vi "LOC subReadWriteVIStringINIKeys(Boolean).vi"(4 "Mode":enum16{"Read", "Write"}(ring), 5 "Section":string, 6 "error in (no error)":errorcluster, 8 "ConfigFileRefnum":T1, 9 "ControlRefnum":refnum<vi>) -> (0 "error out":errorcluster)   [LabVIEW 2020, in "Localization_Tools.lvlib"]
uses:
  Localization_Tools.lvlib
  <vilib>/Utility/config.llb/Config Data RefNum.ctl
  <vilib>/Utility/config.llb/NI_LVConfig.lvlib
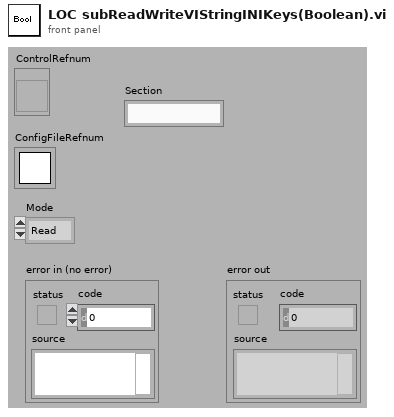
[diagram p1: front panel]
types:
  T1 = typedef "NI_LVConfig.lvlib/Config Data RefNum.ctl" = refnum<k1>
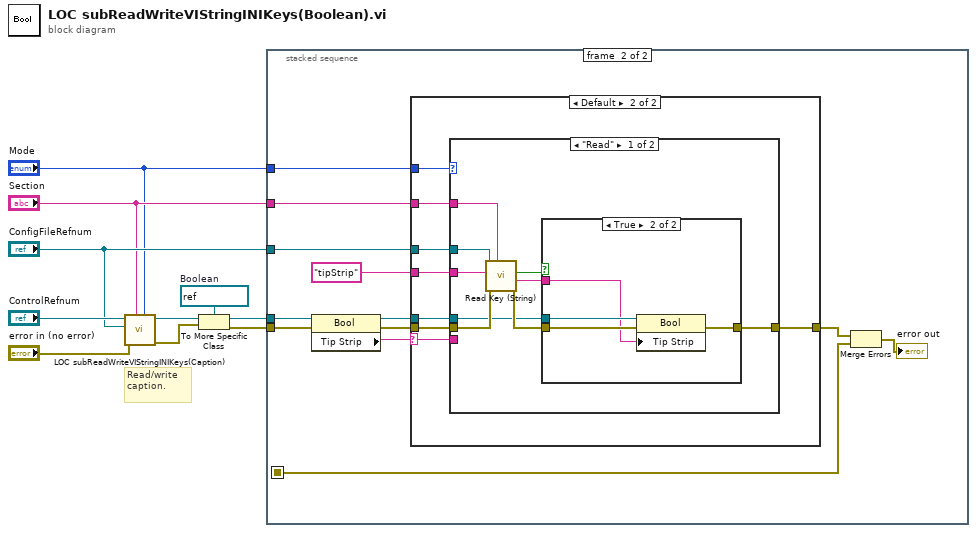
[diagram p0: block diagram]
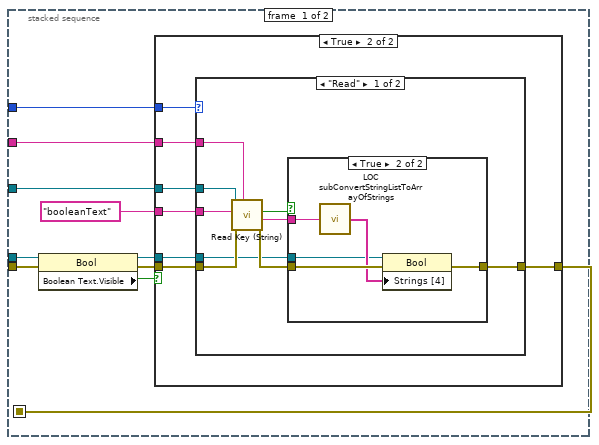
[diagram p2: hidden frame]
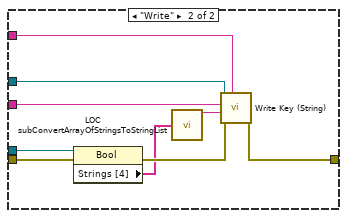
[diagram p5: hidden frame]
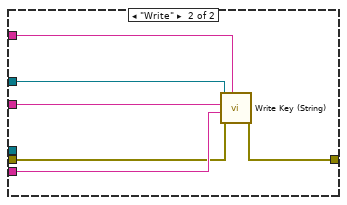
[diagram p8: hidden frame]
diagram:
  w5 = refnum<vi> refnum  # Boolean
  # "Read/write\ncaption."
  n1 = call "LOC subReadWriteVIStringINIKeys(Caption).vi"("Mode"="Mode", "Section"="Section", "error in (no error)"="error in (no error)", "ConfigFileRefnum"="ConfigFileRefnum", "ControlRefnum"="ControlRefnum") -> ("error out"=w3:errorcluster, "dup ControlRefnum"=w4:refnum<vi>)  [unwired: 3 in]
  n2 = To More Specific Class(target class=w5, reference=w4, error in=w3) -> (specific class reference=w2:refnum<vi>, error out=w1:errorcluster)
  n3 = stacked-sequence {
    seq-local: [w12 _] -> [_ w54]
    tunnel: "ConfigFileRefnum" -> [w20 w64]
    tunnel: "Section" -> [w19 w63]
    tunnel: "Mode" -> [w18 w62]
    tunnel: w2 -> [w15 w61]
    tunnel: w1 -> [w14 w60]
    frame #0 {
      n4 = property class="Bool"(reference=w15, error in=w14) -> (reference out=w17:refnum<vi>, error out=w16:errorcluster, "Boolean Text.Visible"=w13:bool)
      n5 = case shown="True" w13 {
        tunnel: "booleanText" ("key") -> [_ w28]
        tunnel: w20 -> [_ w27]
        tunnel: w19 -> [_ w26]
        tunnel: w18 -> [_ w25]
        tunnel: [w21 w24] -> w12
        tunnel: w17 -> [_ w23]
        tunnel: w16 -> [w21 w22]
        frame False {
          # "Boolean text not visible, don't need to read/write\nthe ini entry."
        }
        frame True {
          n6 = case shown="\"Read\"" w25 {
            tunnel: w23 -> [w30 w45]
            tunnel: w27 -> [w37 w52]
            tunnel: w26 -> [w36 w50]
            tunnel: w28 -> [w35 w51]
            tunnel: [w33 w48] -> w24
            tunnel: w22 -> [w31 w44]
            frame "Read" {
              n7 = call <vilib>:"Read Key (String).vi"("section"=w36, "error in (no error)"=w31, "key"=w35, "refnum"=w37) -> ("error out"=w34:errorcluster, "value"=w32:string, "found?"=w29:bool)  [unwired: 4 in, 1 out]
              n8 = case shown="True" w29 {
                tunnel: w34 -> [w38 w43]
                tunnel: [w38 w42] -> w33
                tunnel: w32 -> [_ w41]
                tunnel: w30 -> [_ w39]
                frame False {
                }
                frame True {
                  n9 = call "LOC subConvertStringListToArrayOfStrings.vi"("InputString"=w41) -> ("OutputArray"=w40:string[])
                  n10 = property class="Bool"(reference=w39, error in=w43, "Strings [4]"=w40) -> (error out=w42:errorcluster)  [unwired: 1 out]
                }
              }
            }
            frame "Write" {
              n11 = property class="Bool"(reference=w45, error in=w44) -> (error out=w49:errorcluster, "Strings [4]"=w47:string[])  [unwired: 1 out]
              n12 = call "LOC subConvertArrayOfStringsToStringList.vi"("InputArray"=w47) -> ("OutputString"=w46:string)
              n13 = call <vilib>:"Write Key (String).vi"("section"=w50, "error in (no error)"=w49, "value"=w46, "key"=w51, "refnum"=w52) -> ("error out"=w48:errorcluster)  [unwired: 4 in, 2 out]
            }
          }
        }
      }
    }
    frame #1 {
      n14 = property class="Bool"(reference=w61, error in=w60) -> (reference out=w56:refnum<vi>, error out=w57:errorcluster, "Tip Strip"=w59:string)
      n15 = case shown="Default" w59 {
        selector: w59 -> [_ w68]
        tunnel: "tipStrip" ("key") -> [_ w73]
        tunnel: w64 -> [_ w72]
        tunnel: w63 -> [_ w71]
        tunnel: w62 -> [_ w70]
        tunnel: [w65 w69] -> w55
        tunnel: w57 -> [w65 w67]
        tunnel: w56 -> [_ w66]
        frame "" {
          # "no tipstrip, don't need to read/write\nthe ini entry."
        }
        frame Default {
          n16 = case shown="\"Read\"" w70 {
            tunnel: w72 -> [w82 w93]
            tunnel: w71 -> [w81 w91]
            tunnel: w73 -> [w80 w92]
            tunnel: [w78 w90] -> w69
            tunnel: w67 -> [w76 w88]
            tunnel: w68 -> [_ w89]
            tunnel: w66 -> [w74 _]
            frame "Read" {
              n17 = call <vilib>:"Read Key (String).vi"("section"=w81, "error in (no error)"=w76, "key"=w80, "refnum"=w82) -> ("error out"=w79:errorcluster, "value"=w77:string, "found?"=w75:bool)  [unwired: 4 in, 1 out]
              n18 = case shown="True" w75 {
                tunnel: w79 -> [w83 w87]
                tunnel: [w83 w86] -> w78
                tunnel: w77 -> [_ w84]
                tunnel: w74 -> [_ w85]
                frame False {
                }
                frame True {
                  n19 = property class="Bool"(reference=w85, error in=w87, "Tip Strip"=w84) -> (error out=w86:errorcluster)  [unwired: 1 out]
                }
              }
            }
            frame "Write" {
              n20 = call <vilib>:"Write Key (String).vi"("section"=w91, "error in (no error)"=w88, "value"=w89, "key"=w92, "refnum"=w93) -> ("error out"=w90:errorcluster)  [unwired: 4 in, 2 out]
            }
          }
        }
      }
      n21 = Merge Errors(w55, w54) -> (→"error out":errorcluster)
    }
  }
